vi "Enqueue (Array).vi"(4 "timeout in ms (-1)":i32=-1, 6 "Priority Message? Array":bool[](array[boolean]), 8 "error in (no error)":errorcluster, 9 "Message Data Array":variant[](array[variant]), 10 "States":T2[](array[typedef]), 11 "Message Queue":T1) -> (0 "error out":errorcluster, 3 "Message Queue dub":T1)   [LabVIEW 2019, in "Acquire Mouse.lvlib"]
doc: "For a regular message, enqueue the message. For a priority message, enqueue it at the front of the queue."
uses:
  Acquire Mouse.lvlib
  State Name.ctl
  Shared/TypeDefs/Message Queue Ref.ctl
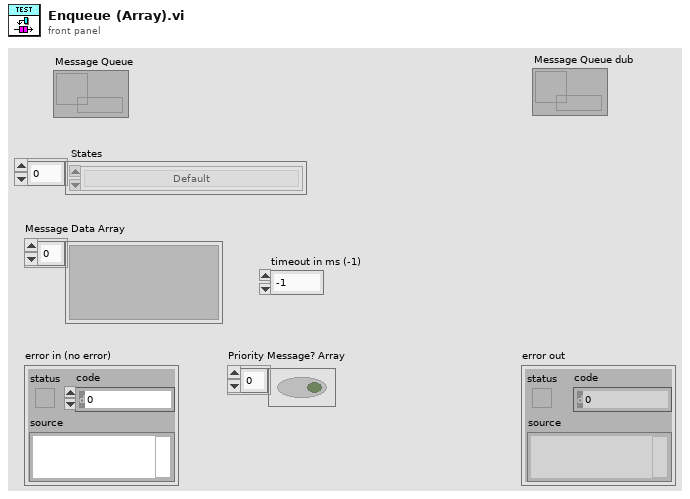
[diagram p1: front panel]
types:
  T1 = typedef "Message Queue Ref.ctl" = refnum<queue>
  T2 = typedef "Acquire Mouse.lvlib/State Name.ctl" = enum16{"Initialize", "Re-Initialize", "Initialize Data", "Initialize Panel", "[Event Structure] Update Data", "Add VI", "Get Splitters", "Map Splitter Pos to Coords", "Initialize Mouse", "Acquire Data", "Process Data", "Error", "Exit", "Default"}
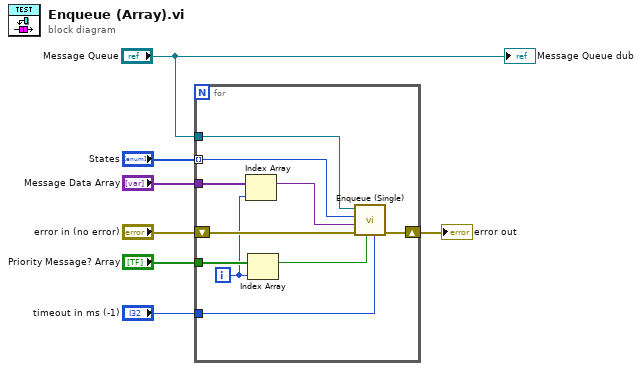
[diagram p0: block diagram]
diagram:
  n1 = for {
    tunnel: "Message Data Array" -> [w15]
    tunnel: "Priority Message? Array" -> [w16]
    tunnel: "Message Queue" -> [w13]
    shift-right: [w11] -> w4
    shift-left: "error in (no error)" -> [w17]
    tunnel: "States" -> [w14] mode=indexing
    tunnel: "timeout in ms (-1)" -> [w12]
    i -> [w8]
    n2 = Index Array(array=w15, index=w8) -> (element=w10:variant)
    n3 = Index Array(array=w16, index=w8) -> (element=w9:bool)
    n4 = call "Enqueue (Single).vi"("timeout in ms (-1)"=w12, "Priority Message? Array"=w9, "error in (no error)"=w17, "Message Data Array"=w10, "States"=w14, "Message Queue"=w13) -> ("error out"=w11:errorcluster)  [unwired: 4 in, 1 out]
  }
  "error out" <- w4
  "Message Queue dub" <- "Message Queue"
